vi "SENS_CORR_COLL_ACQ_POW.vi"(0 "VISA IN":refnum<visa-resource-name>="GPIB0::16::INSTR", 1 "Class":string, 2 "SubClass":string, 5 "error in":errorcluster, 7 "Channel":i32=1) -> (14 "VISA Out":refnum<visa-resource-name>, 19 "error out":errorcluster)   [LabVIEW 2018, in "PNA-X.lvlib"]
doc: "SENSe<cnum>:CORRection:COLLect[:ACQuire] <class>[,subclass] \n(Write-only) For UNGUIDED calibration, measures the specified standards from the selected \ncalibration kit. The calibration kit is selected using the Sense:Correction:Collect:CKIT command. \nFor using two sets of standards, see SENS:CORR:TST. \nNote: Before using this command you must select two items: \n1. Select a calibration method using SENS:CORR:COLL:METH \n2. Select a measurement using CALC:PAR:SEL. You can select one measurement for each channel. \nParameters \n<cnum> Any existing channel number. If unspecified, value is set to 1 \n<class> Measures the standards associated with these class labels. Choose from: \n1626\n\nLabel Forward Reverse \nSTAN1 S11A S22A \nSTAN2 S11B S22B \nSTAN3 S11C S22C \nSTAN4 S21T S12T \nSTAN5 Generic Isolation; not associated with calibration kit definition. \nECAL1 \nthrough \nECAL8 \nECAL modules \nPOWer Take a receiver power cal sweep and turn correction ON \nSLSET Sets 'sliding load type', and increments the \"number of slides\" count. \nThe total number of slides is critical to the correct calculation of the \nsliding load algorithm. See a sliding load cal example. \nSLDONE Computes the sliding load using a circle fit algorithm. \n[subclass] Optional argument. For mechanical calibration kits, choose from the following to \nspecify the standard to be acquired from the SENS:CORR:COLL:CKIT:ORDer list. \nIf not specified, subclass is set to SST1. \nSST1 First standard in the order list \nSST2 Second standard in the order list \nSST3 Third standard in the order list \nSST4 Fourth standard in the order list \nSST5 Fifth standard in the order list \nSST6 Sixth standard in the order list \nSST7 Seventh standard in the order list \nIf an ECAL module (1 through 8) is specified for <class>, choose one of the \nfollowing for specifying which characterization within the ECal module will be \nused for the acquire. If not specified, the default is CHAR0. \nCHAR0 Factory characterization (data that was stored in the ECal module by \nAgilent) \nCHAR1 User characterization #1 \nCHAR2 User characterization #2 \nCHAR3 User characterization #3 \nCHAR4 User characterization #4 \nCHAR5 User characterization #5 \n1627\n\nExamples SENS:CORR:COLL STAN1 \n'If SENS:CORR:COLL:CKIT:ORDer2 5,3,7 \nwas specified, the following command measures standard 3 (the \nsecond in the order list) \nsense1:correction:collect:acquire stan3,sst2 \nSENS:CORR:COLL ECAL4 \nsense2:correction:collect:acquire ecal2,char1 \nQuery Syntax Not applicable \nDefault Not applicable"
uses:
  PNA-X.lvlib
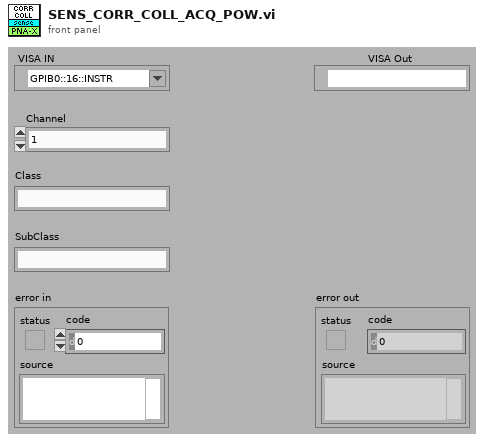
[diagram p1: front panel]
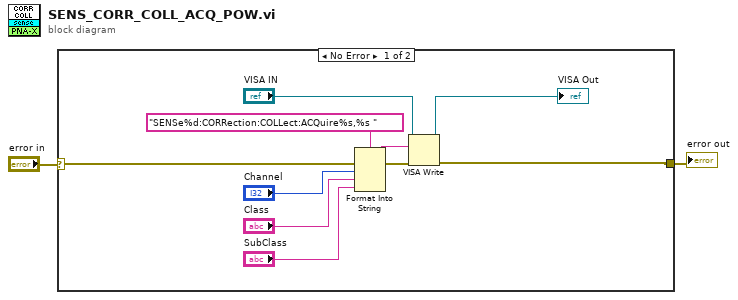
[diagram p0: block diagram]
diagram:
  n1 = case shown="No Error" "error in" {
    selector: "error in" -> [w12 w13]
    tunnel: [w7 w13] -> w1
    frame No Error {
      n2 = Format Into String(format string="SENSe%d:CORRection:COLLect:ACQuire%s,%s " ("Cmdline"), error in=w12, "Channel", "Class", "SubClass") -> (resulting string=w10:string, error out=w11:errorcluster)  [unwired: 1 in]
      n3 = VISA Write(VISA resource name="VISA IN", write buffer=w10, error in (no error)=w11) -> (VISA resource name out=→"VISA Out":refnum<visa-resource-name>, error out=w7:errorcluster)  [unwired: 1 out]
    }
    frame Error {
    }
  }
  "error out" <- w1
